vi "DCWriteXTemplateJK2.vi"(3 ";error in (no error)":errorcluster, 5 ";Type":i32, 6 ";DataIn":string) -> (0 "error IO":errorcluster, 1 "Timestamp dummy":T1 {"ID" format="%x"}, 2 ";Data out":string)   [LabVIEW 2017]
uses:
  <vilib>/variable/detnetvar/Network provider/DC2.llb/DCTerminalRefNum.ctl
  <vilib>/variable/detnetvar/DSV init parameters.ctl
  <vilib>/variable/detnetvar/Network provider/lvedc.dll
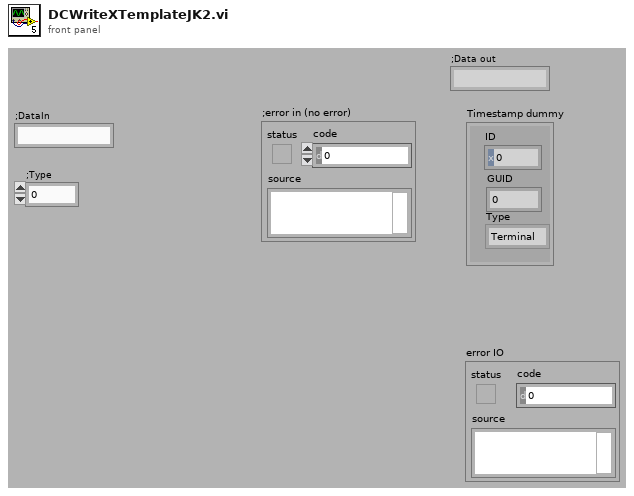
[diagram p1: front panel]
types:
  T1 = typedef "DCTerminalRefNum.ctl" = cluster{"ID":i32, "GUID":dbl, "Type":enum16{"Terminal"}}
  T2 = typedef "DSV init parameters.ctl" = cluster{"refIndex in":i32, "MAC Address":string, "NodeId":string, "SMB block Offset (us)":i32, "Max Variable Length":i32, "Sub Items":i32, "Item Size (bytes)":u16, "Index":i32, "SMB item Data Offset (bytes)":i32, "Timing Source Name":string, "Node is owner?":bool, "Num Items":i32, "Start Slot (us) ":i32, "GUID":string, "Reserved":string, "Cycle time (us)":i32, "Master?":bool, "Max Overall\n Message Length ":i32, "Version Count":u32, "SMB Start Times (other nodes)":i32[], "Network Speed":enum16{"100 MBit", "1 GBit"}, "SMB Variable":bool}
  T3 = typedef "DCTerminalAccessData.ctl" = cluster{"Dif":i32, "Len":i32, "User data":u32}
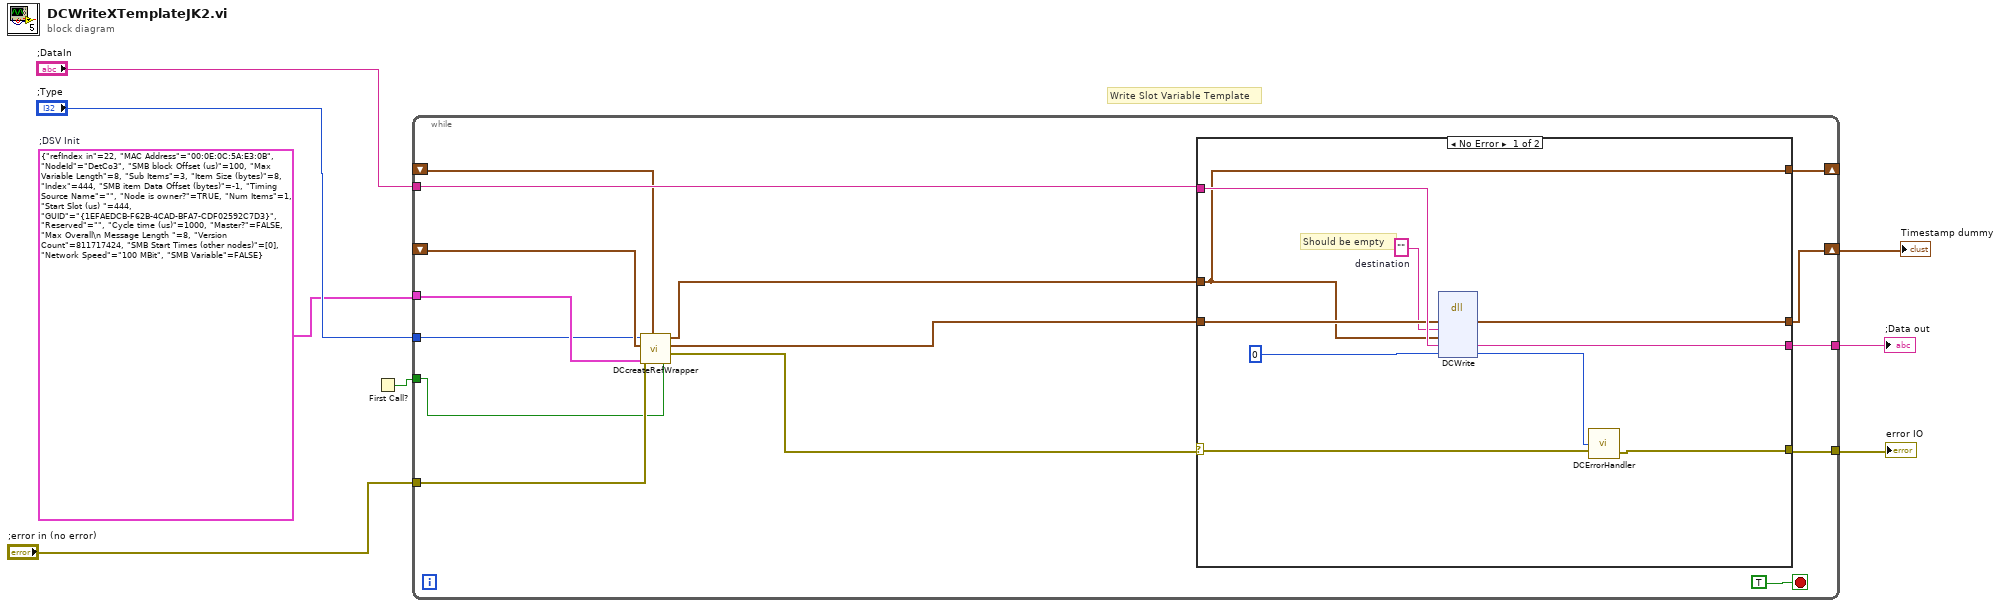
[diagram p0: block diagram]
diagram:
  w1 = T2 {"refIndex in"=22, "MAC Address"="00:0E:0C:5A:E3:0B", "NodeId"="DetCo3", "SMB block Offset (us)"=100, "Max Variable Length"=8, "Sub Items"=3, "Item Size (bytes)"=8, "Index"=444, "SMB item Data Offset (bytes)"=-1, "Timing Source Name"="", "Node is owner?"=TRUE, "Num Items"=1, "Start Slot (us) "=444, "GUID"="{1EFAEDCB-F62B-4CAD-BFA7-CDF02592C7D3}", "Reserved"="", "Cycle time (us)"=1000, "Master?"=FALSE, "Max Overall\n Message Length "=8, "Version Count"=811717424, "SMB Start Times (other nodes)"=[0], "Network Speed"=enum."100 MBit", "SMB Variable"=FALSE}  # ;DSV Init
  # "Write Slot Variable Template"
  n1 = First Call?() -> (First Call?: T/F=w5:bool)
  n2 = while {
    tunnel: [w23] -> w6
    tunnel: ";error in (no error)" -> [w13]
    tunnel: ";DataIn" -> [w22]
    tunnel: [w21] -> w7
    shift-right: [w19] -> w8
    shift-left: _ -> [w12]
    tunnel: w5 -> [w10]
    tunnel: w1 -> [w11]
    shift-right: [w18] -> _
    shift-left: _ -> [w17]
    tunnel: ";Type" -> [w9]
    stop <- TRUE stop-if-true
    n3 = call <vilib>:"DCcreateRefWrapper.vi"("First Call?: T/F"=w10, ";Init"=w11, ";Terminal Data in"=w17, ";error in (no error)"=w13, "Terminal RefNum (out)"=w12, ";Type"=w9) -> ("Error (out)"=w14:errorcluster, "Terminal RefNum (out) 2"=w15:T1, ";Terminal Data"=w16:T3)  [unwired: 1 in]
    n4 = case shown="No Error" w14 {
      selector: w14 -> [w26 w36]
      tunnel: [w27 w36] -> w23
      tunnel: [w33 w37] -> w19
      tunnel: w16 -> [w24 w34]
      tunnel: w22 -> [w32 w35]
      tunnel: w15 -> [w31 w37]
      tunnel: [w30 w35] -> w21
      tunnel: [w24 w34] -> w18
      frame No Error {
        w29 = ""  # destination
        # "Should be empty"
        n5 = dll-call lib="e:/penguin/lvdist/win32/export/17.0/17.0.0f0/dist/vi.lib/variable/detnetvar/Network provider/lvedc.dll" fn="DCWrite"("Terminal RefNum (out) 2"=w31, "destination"=w29, ";Terminal Data"=w24, ";DataIn"=w32, "status"=0) -> ("Terminal RefNum (out) 2"=w33:T1, ";DataIn"=w30:string, "status"=w25:i32)  [unwired: 6 in, 2 out]
        n6 = call <vilib>:"DCErrorHandler.vi"("error in"=w26, "status"=w25) -> ("error out"=w27:errorcluster)  [unwired: 2 in]
      }
      frame Error {
      }
    }
  }
  "Timestamp dummy" <- w8
  ";Data out" <- w7
  "error IO" <- w6
